vi "api_get.vi"() -> ()   [LabVIEW 2020]
uses:
  <vilib>/httpClient/LabVIEWHTTPClient.lvlib
panel:
  out "Full URL":string
  in  "API Key":string="Denver"
  in  "City Name":string="Denver"
  out "body":string
  out "headers":string
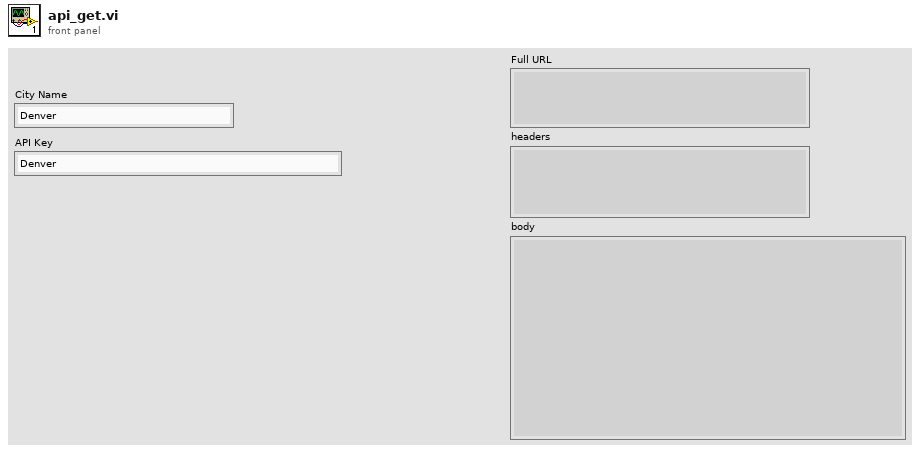
[diagram p1: front panel]
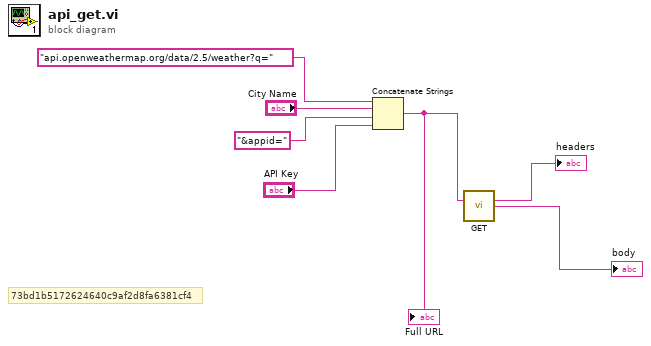
[diagram p0: block diagram]
diagram:
  # "73bd1b5172624640c9af2d8fa6381cf4"
  n1 = Concatenate Strings("api.openweathermap.org/data/2.5/weather?q=", "City Name", "&appid=", "API Key") -> (w1:string)
  "Full URL" <- w1
  n2 = call <vilib>:"GET.vi"("url"=w1) -> ("headers"=→"headers":string, "body"=→"body":string)  [unwired: 11 in, 2 out]
